vi "Drive Controller.vi"(8 "error in":errorcluster) -> ()   [LabVIEW 2017]
doc: "This VI executes continuously carrying out the current operation and responding to updates or new operation requests. It will often contain the timing or control code that is difficult to place directly in TeleOp. This VI generally opens all sensors and motors and isolates the rest of the robot code from knowing implementation details of how the operations are carried out."
uses:
  Drive Operations.ctl
  Drive Setpoints.ctl
  <vilib>/Rock Robotics/WPI/SafetyOutput/WPI_SafetyOutputConfigMenu.ctl
  <vilib>/Rock Robotics/WPI/RobotDrive/WPI_RobotDriveOpen2MotorWithExistingMotors.vi
  <vilib>/Rock Robotics/WPI/Framework/Completion Status.ctl
panel:
  in  "Interactive Values":T1
  in  "Buttons":cluster{"Execute Cmd":bool, "Abort Cmd":bool}
  out "Command Timing":cluster{"Start Time (ms)":u32, "Iterations":i32}
  out "Status":T3
  out "Setpoints":T4(graph)
  out "Current\nCmd":string
  # "Tip: The graph shows the motor setpoints. It may also be helpful to observe inputs and sensor values.\nYou may also want to display tuning or debugging controls."
  # "Interactive Command: You may fill in the settings for a command\nand schedule it with the Execute button. You can observe and abort\nany command while fine tuning the code for the controller."
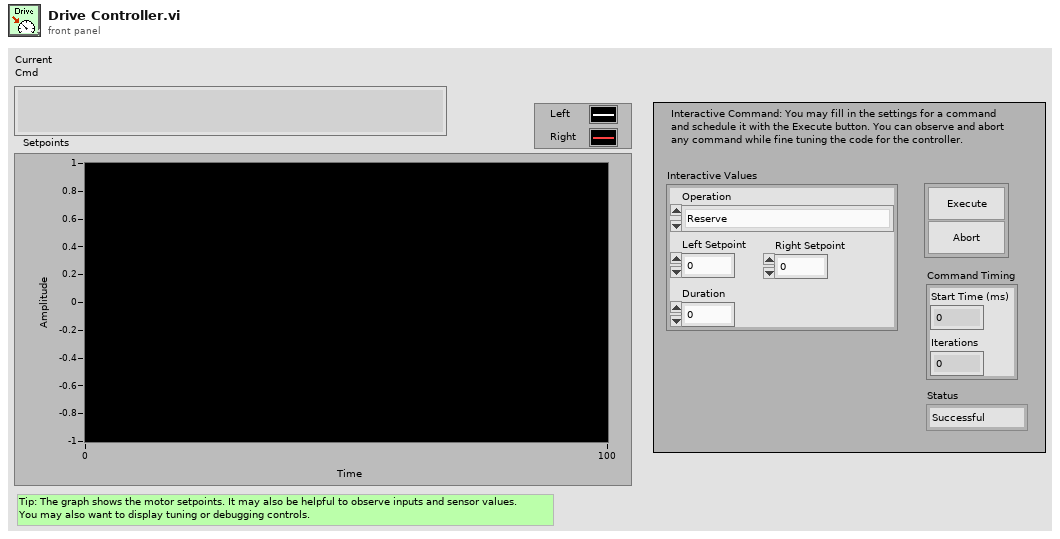
[diagram p1: front panel]
types:
  T1 = typedef "Drive Setpoints.ctl" = cluster{"Operation":T2, "Left Setpoint":dbl, "Right Setpoint":dbl, "Duration":dbl}
  T2 = typedef "Drive Operations.ctl" = enum16{"Reserve", "Read Current", "Immediate", "Drive for Time", "Drive for Distance"}
  T3 = typedef "Completion Status.ctl" = enum16{"Successful", "Aborted", "Incomplete"}
  T4 = cluster{"Left Setpoint":dbl, "Right Setpoint":dbl}
  T5 = typedef "WPI_SafetyOutputConfigMenu.ctl" = enum16{"Enable", "Disable"}
  T6 = typedef "WPI_MotorControlDeviceRef.ctl" = cluster{"DeviceStatus":errorcluster, "Type":T7, "PWM":cluster{"PWM Channel":T8, "DeadBand":T9}, "CAN":cluster{"Device Number":u8, "SetOutput VI Ref":variant, "GetOutput VI Ref":variant, "Enable VI Ref":variant, "Disable VI Ref":variant, "Data":variant}, "Invert":bool, "DIO PWM":cluster{"PWM \"Enable\" Channel":T8, "DIOChannel":T10, "PWM Rate":dbl}}
  T7 = typedef "WPI_MotorControlType.ctl" = enum16{"PWM", "CAN", "DIO PWM"}
  T8 = typedef "FPGA_DIOPWMChannel.ctl" = enum8{"PWM 0", "PWM 1", "PWM 2", "PWM 3", "PWM 4", "PWM 5", "PWM 6", "PWM 7", "PWM 8", "PWM 9", "PWM MXP 0", "PWM MXP 1", "PWM MXP 2", "PWM MXP 3", "PWM MXP 4", "PWM MXP 5", "PWM MXP 6", "PWM MXP 7", "PWM MXP 8", "PWM MXP 9", "Invalid"}
  T9 = typedef "WPI_PWMDeadband.ctl" = cluster{"Name":string, "maxPositivePwm":i32, "minPositivePwm":i32, "centerPwm":i32, "maxNegativePwm":i32, "minNegativePwm":i32, "angularRange":u16}
  T10 = typedef "FPGA_DIOChannel.ctl" = enum8{"DIO 0", "DIO 1", "DIO 2", "DIO 3", "DIO 4", "DIO 5", "DIO 6", "DIO 7", "DIO 8", "DIO 9", "DIO MXP 0", "DIO MXP 1", "DIO MXP 2", "DIO MXP 3", "DIO MXP 4", "DIO MXP 5", "DIO MXP 6", "DIO MXP 7", "DIO MXP 8", "DIO MXP 9", "DIO MXP 10", "DIO MXP 11", "DIO MXP 12", "DIO MXP 13", "DIO MXP 14", "DIO MXP 15", "SPI Port CS1", "SPI Port CS2", "SPI Port CS3", "SPI Port MISO", "SPI Port MOSI", "Invalid"}
  T11 = typedef "WPI_RobotDriveDevRef.ctl" = cluster{"DevStatus":errorcluster, "Motors[]":T6[], "Square Inputs":bool, "Max Output":dbl}
  T12 = typedef "Command Status Info.ctl" = cluster{"Name":string, "Status":T3, "notifier out":T13}
  T13 = typedef "Completion Notifier.ctl" = refnum<notifier>
  T14 = cluster{"SubSystem Data":T1, cluster{"Start Time (ms)":u32, "Iterations":i32}, cluster{"Command Info":T12, "Description":string, "Default Command":T1, "queue out":refnum<queue>, "Subsystem Name":string}}
  T15 = cluster{"SubSystem Data":T1, cluster{"Start Time (ms)":u32, "Iterations":i32}, "Default Command Arguments":cluster{"Command Info":T12, "Description":string, "Default Command":T1, "queue out":refnum<queue>, "Subsystem Name":string}}
  T16 = cluster{"Don't move motors while reserved":dbl, "Don't move motors while reserved":dbl}
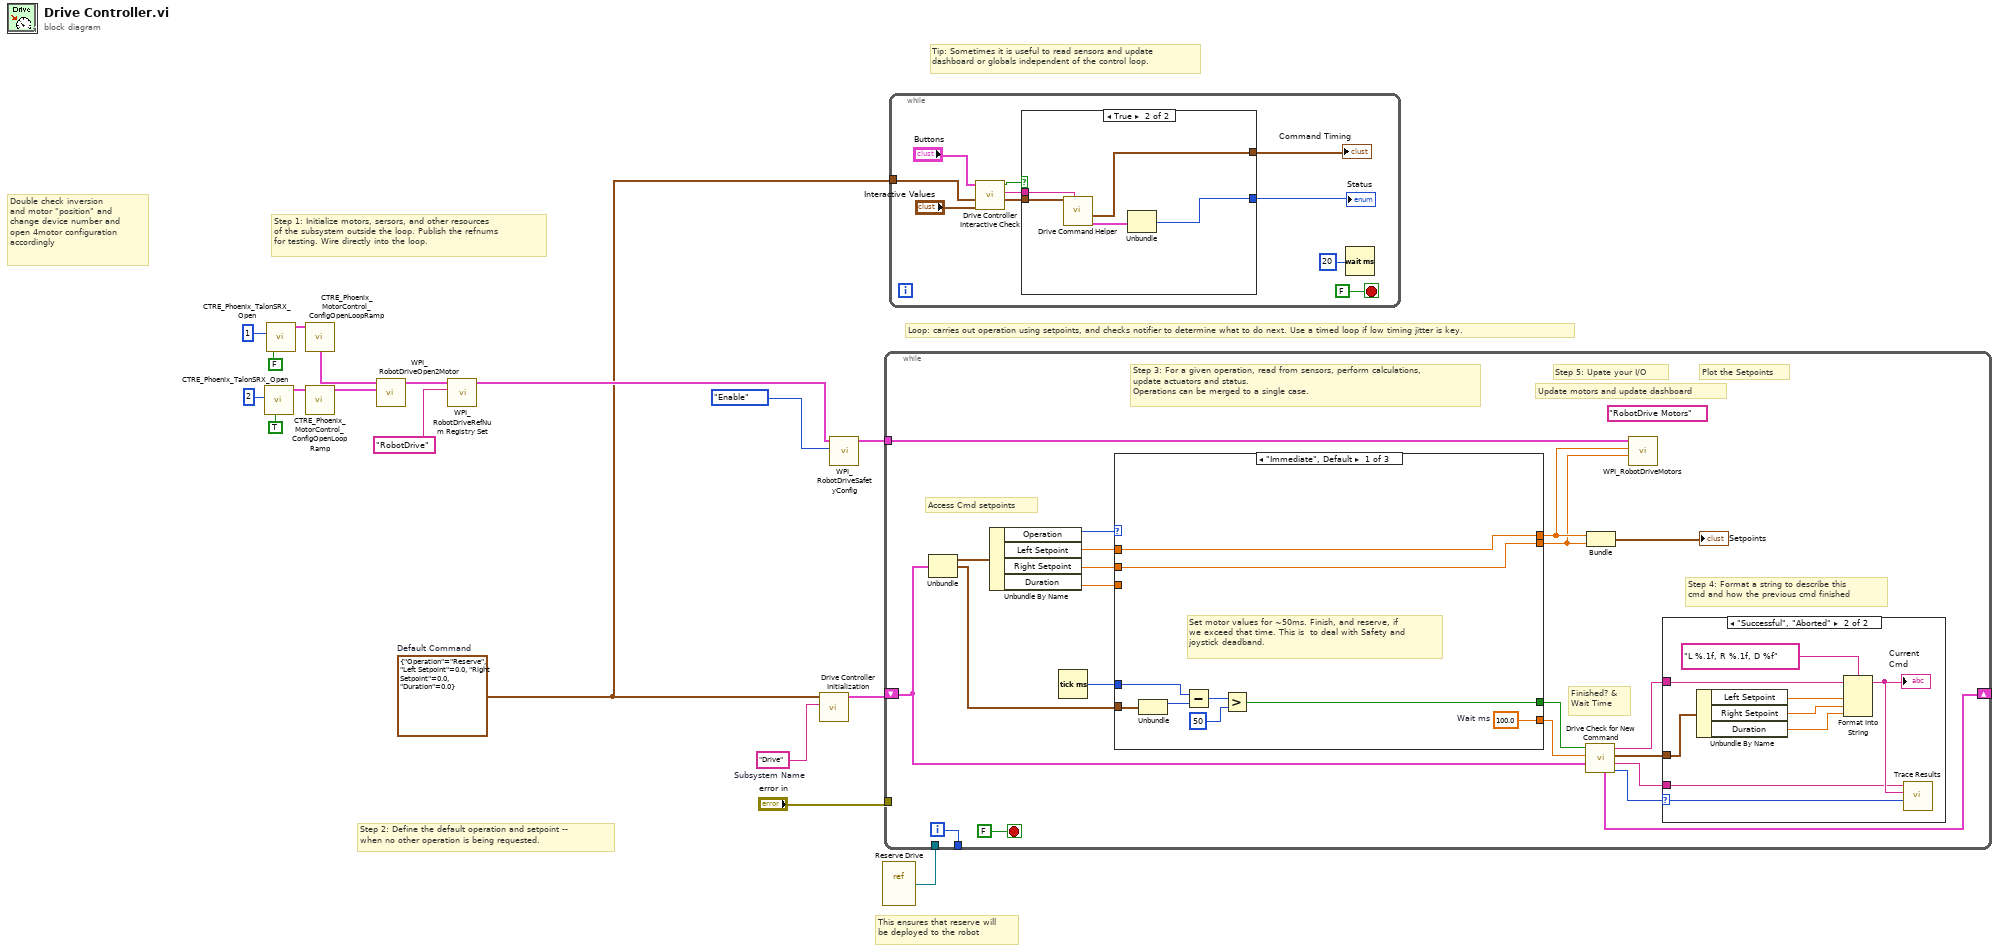
[diagram p0: block diagram]
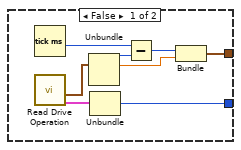
[diagram p2: hidden frame]
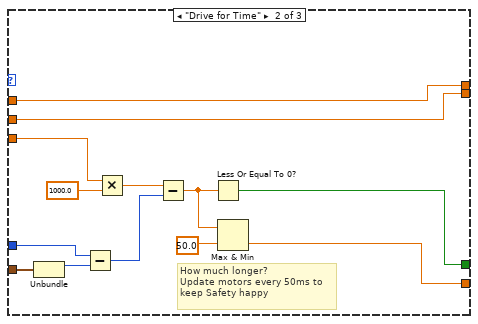
[diagram p4: hidden frame]
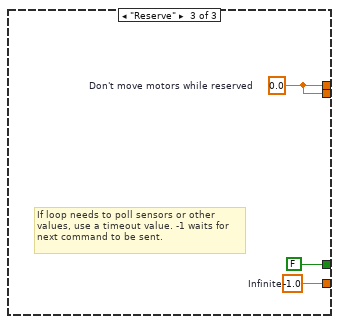
[diagram p5: hidden frame]
diagram:
  w11 = T1 {"Operation"=enum."Reserve", "Left Setpoint"=0.0, "Right Setpoint"=0.0, "Duration"=0.0}  # Default Command
  w18 = "Drive"  # Subsystem Name
  # "Double check inversion\nand motor \"position\" and\nchange device number and \nopen 4motor configuration\naccordingly"
  # "This ensures that reserve will\nbe deployed to the robot"
  # "Tip: Sometimes it is useful to read sensors and update\ndashboard or globals independent of the control loop."
  # "Step 2: Define the default operation and setpoint --\nwhen no other operation is being requested."
  # "Step 1: Initialize motors, sersors, and other resources\nof the subsystem outside the loop. Publish the refnums\nfor testing. Wire directly into the loop."
  # "Loop: carries out operation using setpoints, and checks notifier to determine what to do next. Use a timed loop if low timing jitter is key."
  n1 = call <vilib>:"CTRE_Phoenix_TalonSRX_Open.vi"("Invert"=TRUE, "Device Number"=u8 2) -> ("CAN Talon SRX Ref"=w9:T6)  [unwired: 8 in, 1 out]
  n2 = call <vilib>:"CTRE_Phoenix_TalonSRX_Open.vi"("Invert"=FALSE, "Device Number"=u8 1) -> ("CAN Talon SRX Ref"=w10:T6)  [unwired: 8 in, 1 out]
  n3 = call <vilib>:"CTRE_Phoenix_MotorControl_ConfigOpenLoopRamp.vi"("PhoenixMotorControlDevRef"=w10) -> ("PhoenixMotorControlDevRef"=w3:T6)  [unwired: 9 in, 1 out]
  n4 = call <vilib>:"CTRE_Phoenix_MotorControl_ConfigOpenLoopRamp.vi"("PhoenixMotorControlDevRef"=w9) -> ("PhoenixMotorControlDevRef"=w2:T6)  [unwired: 9 in, 1 out]
  n5 = call-poly <vilib>:"WPI_RobotDriveOpen2Motor.vi"("Right Motor Dev Ref"=w2, "Left Motor Dev Ref"=w3) -> ("RobotDriveDevRef"=w1:T11)  [unwired: 8 in, 1 out]
  n6 = call <vilib>:"WPI_RobotDriveRefNum Registry Set.vi"("refnum name"="RobotDrive", "RobotDriveDevRef"=w1) -> ("RobotDriveDevRef"=w17:T11)  [unwired: 2 in, 7 out]
  n7 = call "Drive Controller Initialization.vi"("Subsystem Name"=w18, "Default Command"=w11) -> ("Current Command"=w13:T14)  [unwired: 9 in]
  n8 = call <vilib>:"WPI_RobotDriveSafetyConfig.vi"("mode"=WPI_SafetyOutputConfigMenu."Enable", "RobotDriveDevRef"=w17) -> ("RobotDriveDevRef"=w15:T11)  [unwired: 8 in, 1 out]
  n9 = vi-ref "Reserve Drive.vi"() -> (w12:refnum<vi>)
  n10 = while {
    shift-right: [w26] -> _
    shift-left: w13 -> [w19]
    tunnel: [w38] -> _
    tunnel: w15 -> [w34]
    tunnel: "error in" -> [_]
    tunnel: w12 -> [_]
    i -> [w38]
    stop <- FALSE stop-if-true
    (unwired) "RobotDrive Motors" ("Name")
    # "Step 5: Upate your I/O"
    # "Step 4: Format a string to describe this\ncmd and how the previous cmd finished"
    # "Current Command"
    # "Update motors and update dashboard"
    # "Plot the Setpoints"
    # "Access Cmd setpoints"
    # "Finished? &\nWait Time"
    # "Step 3: For a given operation, read from sensors, perform calculations,\nupdate actuators and status.\nOperations can be merged to a single case."
    n11 = Unbundle(w19) -> ("SubSystem Data"=w33:T1, w20:cluster{"Start Time (ms)":u32, "Iterations":i32})  [unwired: 1 out]
    n12 = Unbundle By Name(w33) -> ("Operation"=w32:T2, "Left Setpoint"=w31:dbl, "Right Setpoint"=w30:dbl, "Duration"=w29:dbl)
    n13 = Tick Count (ms)() -> (millisecond timer value=w28:u32)
    n14 = case shown="\"Immediate\", Default" w32 {
      tunnel: [w57 w58 w73] -> w25
      tunnel: [w50 w65 FALSE ("ignore previous (F)")] -> w24
      tunnel: w20 -> [w49 w67 _]
      tunnel: [w56 w64 w71] -> w36
      tunnel: [w55 w63 w71] -> w35
      tunnel: w31 -> [w56 w64 _]
      tunnel: w30 -> [w55 w63 _]
      tunnel: w29 -> [_ w62 _]
      tunnel: w28 -> [w51 w61 _]
      frame "Immediate", Default {
        w57 = 100.0  # Wait ms
        # "Set motor values for ~50ms. Finish, and reserve, if\nwe exceed that time. This is  to deal with Safety and\njoystick deadband."
        n15 = Unbundle(w49) -> ("Start Time (ms)"=w52:u32)  [unwired: 1 out]
        n16 = Subtract(x=w51, y=w52) -> (x-y=w53:u32)
        n17 = Greater?(x=w53, y=u8 50 ("Left Motor")) -> (0:w50:bool)
      }
      frame "Drive for Time" {
        # "How much longer?\nUpdate motors every 50ms to\nkeep Safety happy"
        n18 = Unbundle(w67) -> ("Start Time (ms)"=w66:u32)  [unwired: 1 out]
        n19 = Subtract(x=w61, y=w66) -> (x-y=w70:u32)
        n20 = Multiply(x=w62, y=1000.0) -> (x*y=w69:dbl)
        n21 = Subtract(x=w69, y=w70) -> (x-y=w60:dbl)
        n22 = Less Or Equal To 0?(x=w60) -> (x <= 0?=w65:bool)
        n23 = Max & Min(x=w60, y=50.0) -> (min(x,y)=w58:dbl)  [unwired: 1 out]
      }
      frame "Reserve" {
        w71 = 0.0  # Don't move motors while reserved
        w73 = -1.0  # Infinite
        # "If loop needs to poll sensors or other\nvalues, use a timeout value. -1 waits for\nnext command to be sent."
      }
    }
    n24 = call "Drive Check for New Command.vi"("input cluster"=w19, "Wait time (ms)"=w25, "Finished?"=w24) -> ("Completion"=w27:T3, "Subsystem Name"=w21:string, "Current Command"=w22:T1, "Initial Trace String"=w23:string, "Next Command"=w26:T15)  [unwired: 4 in]
    n25 = Bundle("Don't move motors while reserved"=w36, "Don't move motors while reserved"=w35) -> (→"Setpoints":T16)  [unwired: 1 in]
    n26 = call <vilib>:"WPI_RobotDriveMotors.vi"("RightSpeed"=w35, "LeftSpeed"=w36, "RobotDriveDevRef"=w34) -> ()  [unwired: 1 in, 8 out]
    n27 = case shown="\"Successful\", \"Aborted\"" w27 {
      selector: w27 -> [_ w48]
      tunnel: w23 -> [_ w43]
      tunnel: w22 -> [_ w44]
      tunnel: w21 -> [_ w40]
      frame "Incomplete", Default {
        # "Continuing current command"
      }
      frame "Successful", "Aborted" {
        # "Report and setup for next command"
        n28 = Unbundle By Name(w44) -> ("Left Setpoint"=w46:dbl, "Right Setpoint"=w47:dbl, "Duration"=w41:dbl)
        n29 = Format Into String(format string="L %.1f, R %.1f, D %f", initial string=w43, w46, w47, w41) -> (resulting string=w42:string)  [unwired: 1 in, 1 out]
        "Current\nCmd" <- w42
        n30 = call <vilib>:"Trace Results.vi"("Status of previous command"=w48, "Description"=w42, "Subsystem"=w40) -> ()  [unwired: 9 in]
      }
    }
  }
  n31 = while {
    tunnel: w11 -> [w75]
    stop <- FALSE stop-if-true
    n32 = call "Drive Controller Interactive Check.vi"("Interactive Command In"="Interactive Values", "Default Command"=w75, "Buttons"="Buttons") -> ("Interactive Command Out"=w77:T1, "Trace String"=w78:string, "Schedule"=w79:bool)  [unwired: 6 in]
    n33 = case shown="True" w79 {
      tunnel: [w88 w96] -> w80
      tunnel: [w87 w92] -> w81
      tunnel: w78 -> [_ w94]
      tunnel: w77 -> [_ w93]
      frame False {
        n34 = Tick Count (ms)() -> (millisecond timer value=w91:u32)
        n35 = call "Read Drive Operation.vi"() -> ("Command Info"=w85:T12, "SubSystem Data"=w84:T1)  [unwired: 9 in, 1 out]
        n36 = Unbundle(w84) -> ("Operation"=w89:T2, "Left Setpoint"=w86:dbl)  [unwired: 2 out]
        n37 = Unbundle(w85) -> ("Status"=w88:T3)  [unwired: 2 out]
        n38 = Subtract(x=w91, y=w89) -> (x-y=w90:u32)
        n39 = Bundle(w90, "Left Setpoint"=w86) -> (w87:cluster{u32, "Left Setpoint":dbl})  [unwired: 1 in]
      }
      frame True {
        n40 = call "Drive Command Helper.vi"("Description"=w94, "SubSystem Data"=w93) -> ("Command Info Out"=w95:T12, "Command Timing"=w92:cluster{"Start Time (ms)":u32, "Iterations":i32})  [unwired: 7 in, 1 out]
        n41 = Unbundle(w95) -> ("Status"=w96:T3)  [unwired: 2 out]
      }
    }
    "Status" <- w80
    "Command Timing" <- w81
    n42 = Wait (ms)(milliseconds to wait=u32 20) -> ()  [unwired: 1 out]
  }
